vi "Get New Chess Color.vi"(8 "white available position":i32, 9 "black available position":i32, 11 "current color":T1=1) -> (3 "new color":T1=2)   [LabVIEW 2018, in "Othello.xctl"]
doc: "本VI是为《我和LabVIEW》一书编写的示例。\n关于本书的介绍请参考网页：\nhttp://ruanqizhen.spaces.live.com/blog/cns!5852D4F797C53FB6!4310.entry"
uses:
  Othello.xctl
  Control/Pict Ring Chess.ctl
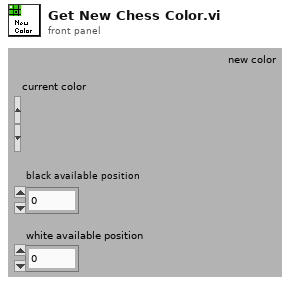
[diagram p1: front panel]
types:
  T1 = typedef "Othello.xctl/Pict Ring Chess.ctl" = u16
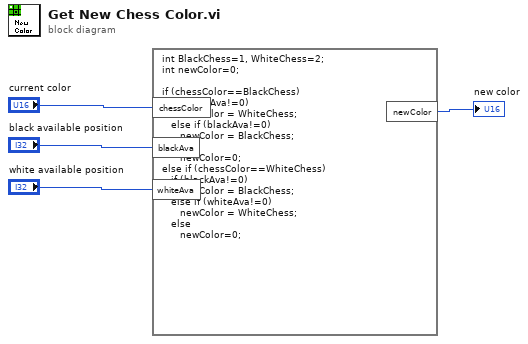
[diagram p0: block diagram]
diagram:
  n1 = formula code="int BlackChess=1, WhiteChess=2;\nint newColor=0;\n\nif (chessColor==BlackChess)\n   if (whiteAva!=0)\n      newColor = WhiteChess;\n   else if (blackAva!=0)\n      newColor = BlackChess;\n   else\n      newColor=0;\nelse if (chessColor==WhiteChess)\n   if (blackAva!=0)\n      newColor = BlackChess;\n   else if (whiteAva!=0)\n      newColor = WhiteChess;\n   else\n      newColor=0;"("chessColor"="current color", "blackAva"="black available position", "whiteAva"="white available position") -> ("newColor"=→"new color":i32)
